vi "20T_Set_Clamp.vi"(8 "error in (no error)":errorcluster, 10 "20T Control":T1={"Clamp"=TRUE, "Switch Heater"=TRUE, "Go to Zero"=TRUE, "Go to Set"=FALSE, "Go to Hold"=FALSE, "Field Setpoint (T)"=3.4572, "Rate Setpoint (T/min)"=0.0, "Set Rate"=FALSE, "Activate lambda control"=FALSE, "Set lambda NV"=FALSE, "lambda NV  SP"=3.4572} {"lambda NV  SP" format="%.1f"; "Rate Setpoint (T/min)" format="%6_5f"; "Field Setpoint (T)" format="%#4_5f"}, 11 "Mercury Reference In":T2) -> (0 "error out":errorcluster)   [LabVIEW 2019]
uses:
  Equipment/Mercury iXX/Public/Controls/Mercury Reference.ctl
  Equipment/Mercury iXX/Public/Controls/Comms Transport Layer.ctl
  Equipment/Mercury iXX/Private/Controls/Query Dynamic Reference.ctl
  Monitor Communication/Gustav/20T_Control.ctl
  Equipment/Mercury iXX/Public/Libraries/Magnet/Open/Open Magnet Device.vi
  Equipment/Mercury iXX/Mercury iXX.lvlib
  Equipment/Mercury iXX/Public/Libraries/Magnet.lvlib
panel:
  # "20 T"
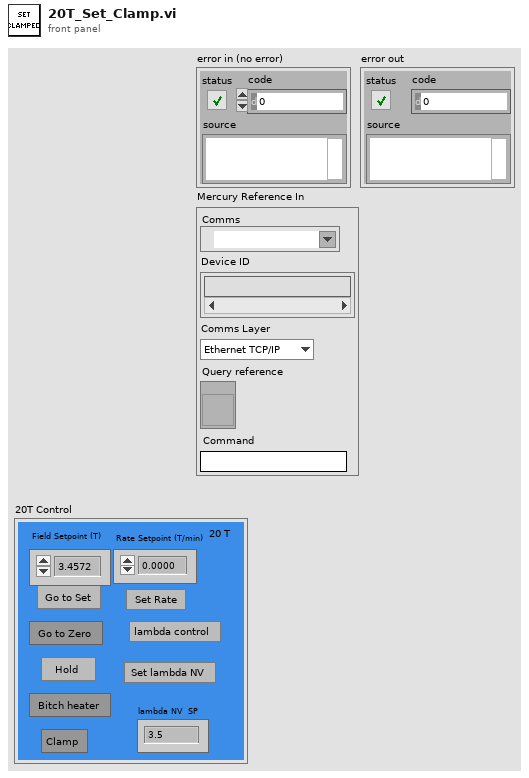
[diagram p1: front panel]
types:
  T1 = typedef "20T_Control.ctl" = cluster{"Clamp":bool, "Switch Heater":bool, "Go to Zero":bool, "Go to Set":bool, "Go to Hold":bool, "Field Setpoint (T)":dbl, "Rate Setpoint (T/min)":dbl, "Set Rate":bool, "Activate lambda control":bool, "Set lambda NV":bool, "lambda NV  SP":dbl}
  T2 = typedef "Mercury iXX.lvlib/Mercury Reference.ctl" = cluster{"Comms":refnum<visa-resource-name>, "Device ID":string[], "Comms Layer":T3, "Command":string, "Query reference":T4}
  T3 = typedef "Mercury iXX.lvlib/Comms Transport Layer.ctl" = enum16{"Ethernet TCP/IP", "USB", "ISOBus - RS-232", "GPIB"}
  T4 = typedef "Mercury iXX.lvlib/Query Dynamic Reference.ctl" = refnum<vi>
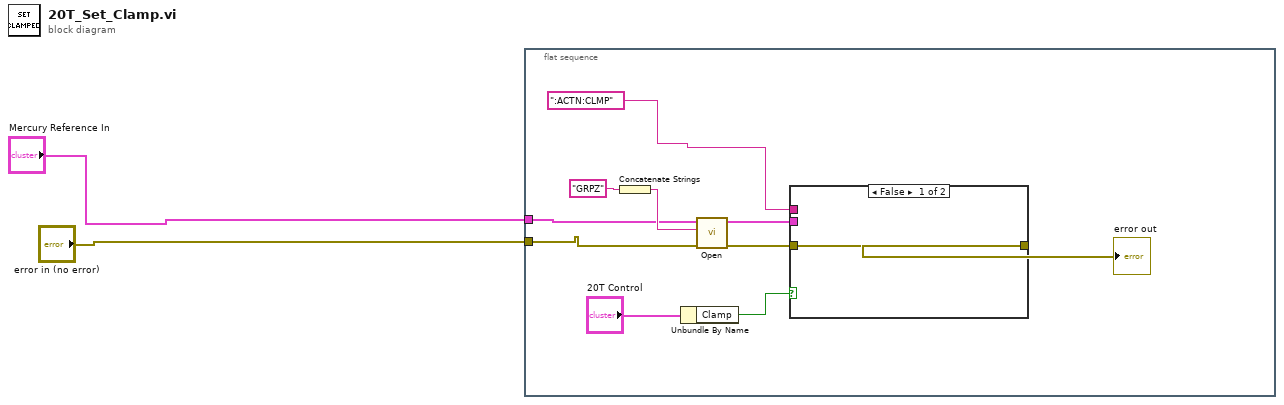
[diagram p0: block diagram]
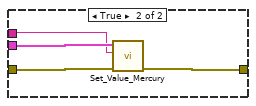
[diagram p2: hidden frame]
diagram:
  n1 = flat-sequence {
    tunnel: "Mercury Reference In" -> [w5]
    tunnel: "error in (no error)" -> [w4]
    frame #0 {
      n2 = Concatenate Strings("GRPZ" ("Device Identifier")) -> (w10:string)
      n3 = Unbundle By Name("20T Control") -> ("Clamp"=w6:bool)
      n4 = call-poly "Open.vi"("error in (no error)"=w4, "Device Identifier"=w10, "Mercury Reference In"=w5) -> ("error out"=w11:errorcluster, "Mercury Reference Out"=w12:T2)  [unwired: 1 in, 6 out]
      n5 = case shown="False" w6 {
        tunnel: w12 -> [_ w17]
        tunnel: w11 -> [w13 w15]
        tunnel: [w13 w16] -> w9
        tunnel: ":ACTN:CLMP" -> [_ w14]
        frame False {
        }
        frame True {
          n6 = call "Set_Value_Mercury.vi"("error in"=w15, "Noun(s)"=w14, "Mercury Reference In"=w17) -> ("error out"=w16:errorcluster)  [unwired: 7 in, 1 out]
        }
      }
      "error out" <- w9
    }
  }
